vi "Periodic Tasks.vi"(8 "error in":errorcluster) -> ()   [LabVIEW 2013]
doc: "This VI runs in parallel to other tasks. It can contain as many user-defined periodic loops as you need. These can carry out PID or other sorts of timed response."
uses:
  RefnameEnum.ctl
  CatchAction.ctl
  CollectorWrapAction.ctl
  ShooterWrapperAction.ctl
  DoubleSolenoidAction.ctl
  SingleSolenoidAction.ctl
  <vilib>/Rock Robotics/SystemInterfaces/Utilities/FPGA_UtilitiesLED Source.ctl
  <vilib>/Rock Robotics/SystemInterfaces/Utilities/FPGA_UtilitiesLED State.ctl
  TankDriveAction.ctl
  SonarAction.ctl
  AutoAlignMode.ctl
  <vilib>/Rock Robotics/WPI/Compressor/WPI_CompressorGetSetRefNum.vi
  Robot Global Data.vi
panel:
  out "AutoDistanceWrapperIterations":i32=4516
  out "AutoDistanceWrapperTimer":u32=21
  in  "Slowdown":dbl=12.0 format="%#_13g"
  in  "Brake":dbl=6.0 format="%#_13g"
  in  "DesiredDistance":dbl=36.0 format="%#_13g"
  out "CatcherWrapperIterations":i32=1817
  out "CatcherWrapperTimer":u32=50
  out "CollectorWrapperTimer":u32=50
  out "CollectorWrapperIterations":i32=1817
  out "ShooterWrapperIterations":i32=1813
  out "ShooterWrapperTimer":u32=50
  out "CollectorIterations":i32=1817
  out "ClapperIterations":i32=1817
  out "RollerPneumaticIterations":i32=1817
  out "RollerMotorIterations":i32=1817
  out "FiringCylinderIterations":i32=1817
  out "KickerIterations":i32=1817
  out "SonicShifterIterations":i32=1817
  out "TankDriveIterations":i32=4509
  out "Collector Timer":u32=50
  out "Clapper Timer":u32=50
  out "Roller Pneumatic Timer":u32=50
  out "Firing Cylinder Timer":u32=50
  out "Sonic Shifter Timer":u32=50
  out "Kicker Timer":u32=50
  out "Roller Motor Timer":u32=50
  out "Tank Drive Timer":u32=21
  # "CATCH"
  # "SHOOTER WRAP"
  # "SONIC SHIFTER"
  # "TANK DRIVE"
  # "COLLECTOR WRAP"
  # "KICKER"
  # "ROLLER MOTOR"
  # "COLLECTOR ARM"
  # "FIRING CYLINDERS"
  # "AUTODISTANCE"
  # "ROLLER PNEUMATIC"
  # "CLAPPER"
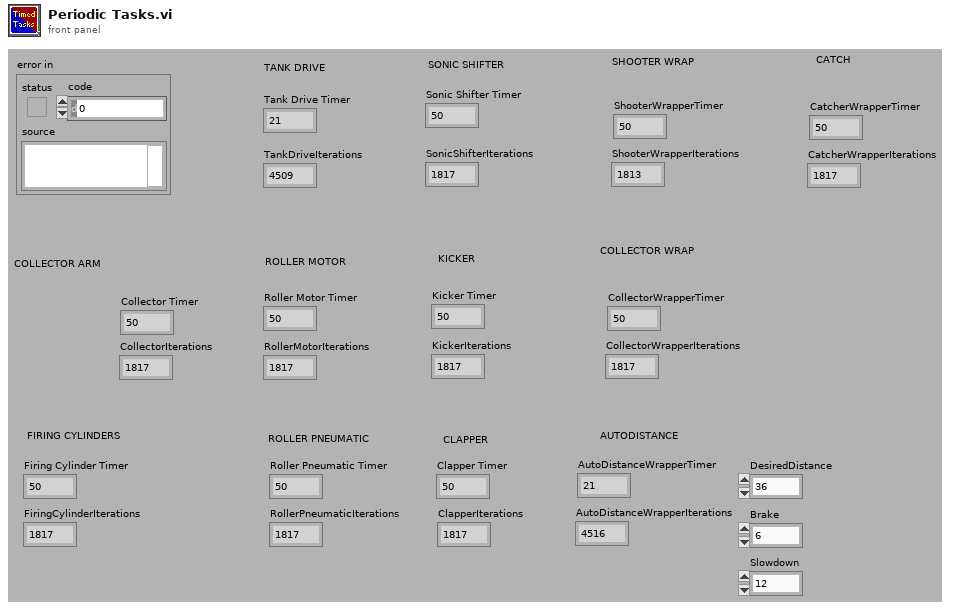
[diagram p1: front panel]
types:
  T1 = typedef "ShooterWrapperAction.ctl" = enum16{"Init", "CollectorDown", "CollectorUp"}
  T2 = typedef "CatchAction.ctl" = enum16{"PreCatch", "Catch", "Stop"}
  T3 = typedef "DoubleSolenoidAction.ctl" = enum16{"Init", "Middle", "In", "Out"}
  T4 = typedef "CollectorAction.ctl" = enum16{"Init", "Raise", "Lower", "Stop", "GetStatus"}
  T5 = typedef "CollectorWrapAction.ctl" = enum16{"PreCollect", "Collect", "Stop"}
  T6 = typedef "SingleSolenoidAction.ctl" = enum16{"Init", "SetState", "Disable"}
  T7 = typedef "TankDriveAction.ctl" = enum16{"Init", "LinearDrive", "SetValue", "Disable"}
  T8 = typedef "AutoAlignMode.ctl" = enum16{"Fullspeed", "Linear"}
  T9 = typedef "SonarAction.ctl" = enum16{"Init", "ReadValue", "Disable"}
  T10 = typedef "FPGA_UtilitiesLED State.ctl" = enum16{"Off", "On", "Toggle"}
  T11 = typedef "FPGA_UtilitiesLED Source.ctl" = enum16{"User LED", "FPGA LED"}
  T12 = typedef "RefnameEnum.ctl" = enum16{"TankDrive", "Controller1", "Controller2", "SonicShifter", "Compressor"}
  T13 = typedef "WPI_CompressorDevRef.ctl" = cluster{"DevStatus":errorcluster, "DigitalInputDevRef":T14, "RelayDevRef":T17}
  T14 = typedef "WPI_DigitalInputDevRef.ctl" = cluster{"DevStatus":errorcluster, "DIO Channel":T15, "Digital Module":T16}
  T15 = typedef "FPGA_DIOChannel.ctl" = enum8{"DIO 1", "DIO 2", "DIO 3", "DIO 4", "DIO 5", "DIO 6", "DIO 7", "DIO 8", "DIO 9", "DIO 10", "DIO 11", "DIO 12", "DIO 13", "DIO 14", "Invalid"}
  T16 = typedef "FPGA_TypedefDigitalModule.ctl" = enum16{"Digital Module 1", "Digital Module 2"}
  T17 = typedef "WPI_RelayDevRef.ctl" = cluster{"DevStatus":errorcluster, "Relay Channel":T18, "Digital Module":T16, "Relay Direction":T19}
  T18 = typedef "FPGA_DIORelayChannel.ctl" = enum8{"Relay 1", "Relay 2", "Relay 3", "Relay 4", "Relay 5", "Relay 6", "Relay 7", "Relay 8", "Invalid"}
  T19 = typedef "WPI_RelayDirection.ctl" = enum16{"Both directions", "Forward only", "Reverse only"}
  T20 = typedef "RollerAction.ctl" = enum16{"Init", "Off", "Forward", "Reverse"}
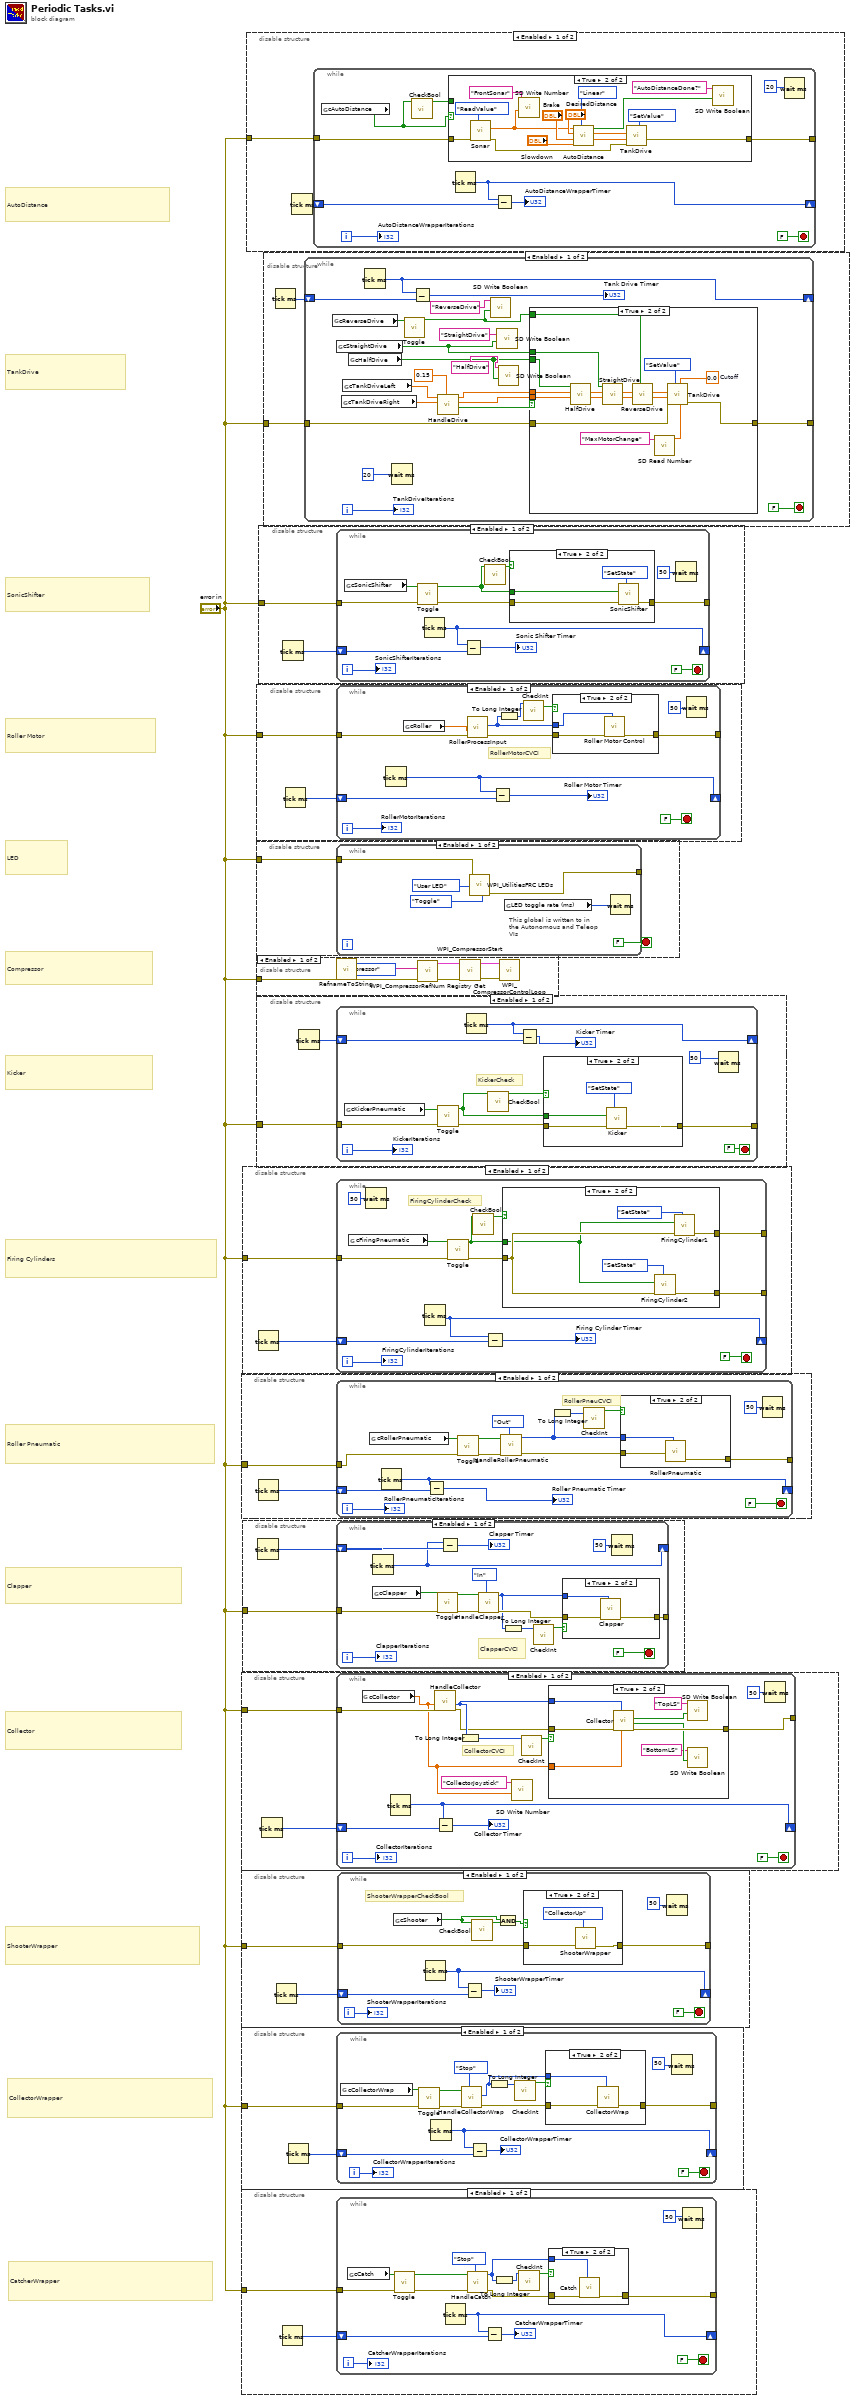
[diagram p0: block diagram]
diagram:
  # "AutoDistance"
  # "CatcherWrapper"
  # "CollectorWrapper"
  # "ShooterWrapper"
  # "Collector"
  # "Clapper"
  # "Roller Pneumatic"
  # "Firing Cylinders"
  # "Kicker"
  # "Compressor"
  # "Roller Motor"
  # "SonicShifter"
  # "LED"
  # "TankDrive"
  n1 = disable-structure shown="Enabled" {
    disable-tunnel: "error in" -> [w3 _]
    frame Enabled {
      n2 = Tick Count (ms)() -> (millisecond timer value=w2:u32)
      n3 = while {
        tunnel: w3 -> [w10]
        shift-right: [w11] -> _
        shift-left: w2 -> [w12]
        tunnel: [w9] -> _
        i -> [w7]
        stop <- FALSE stop-if-true
        # "ShooterWrapperCheckBool"
        n4 = global read "Robot Global Data.vi" "cShooter"() -> (w4:bool)
        n5 = Tick Count (ms)() -> (millisecond timer value=w11:u32)
        n6 = Subtract(x=w11, y=w12) -> (x-y=→"ShooterWrapperTimer":u32)
        n7 = call "CheckBool.vi"("Input Boolean"=w4) -> ("Boolean Changed?"=w6:bool)  [unwired: 10 in]
        n8 = And(x=w4, y=w6) -> (x .and. y?=w5:bool)
        n9 = case shown="True" w5 {
          tunnel: w10 -> [w15 w18]
          tunnel: [w15 w17] -> w9
          frame False {
          }
          frame True {
            n10 = call "ShooterWrapper.vi"("Action"=ShooterWrapperAction."CollectorUp", "error in"=w18) -> ("error out"=w17:errorcluster)  [unwired: 8 in]
          }
        }
        n11 = Wait (ms)(milliseconds to wait=u32 50) -> ()  [unwired: 1 out]
        "ShooterWrapperIterations" <- w7
      }
    }
    frame Disabled {
    }
  }
  n12 = disable-structure shown="Enabled" {
    disable-tunnel: "error in" -> [w20 _]
    frame Enabled {
      n13 = Tick Count (ms)() -> (millisecond timer value=w19:u32)
      n14 = while {
        tunnel: w20 -> [w36]
        tunnel: [w33] -> _
        shift-right: [w28] -> _
        shift-left: w19 -> [w29]
        i -> [w30]
        stop <- FALSE stop-if-true
        n15 = global read "Robot Global Data.vi" "cCatch"() -> (w35:bool)
        n16 = call "Toggle.vi"("error in"=w36, "RawInput"=w35) -> ("error out"=w26:errorcluster, "ToggleState"=w22:bool)  [unwired: 8 in]
        n17 = Tick Count (ms)() -> (millisecond timer value=w28:u32)
        n18 = call "HandleCatch.vi"("InitState"=CatchAction."Stop", "error in (no error)"=w26, "Toggle?"=w22) -> ("error out"=w25:errorcluster, "State"=w23:T2)  [unwired: 7 in]
        n19 = Subtract(x=w28, y=w29) -> (x-y=→"CatcherWrapperTimer":u32)
        n20 = To Long Integer(number=w23) -> (32bit integer=w24:i32)
        n21 = call "CheckInt.vi"("Integer"=w24) -> ("Changed?"=w34:bool)  [unwired: 10 in]
        n22 = case shown="True" w34 {
          tunnel: w25 -> [w37 w40]
          tunnel: [w37 w39] -> w33
          tunnel: w23 -> [_ w38]
          frame False {
          }
          frame True {
            n23 = call "Catch.vi"("Action"=w38, "error in (no error)"=w40) -> ("error out"=w39:errorcluster)  [unwired: 9 in]
          }
        }
        n24 = Wait (ms)(milliseconds to wait=u32 50) -> ()  [unwired: 1 out]
        "CatcherWrapperIterations" <- w30
      }
    }
    frame Disabled {
    }
  }
  n25 = disable-structure shown="Enabled" {
    disable-tunnel: "error in" -> [w42 _]
    frame Enabled {
      n26 = Tick Count (ms)() -> (millisecond timer value=w41:u32)
      n27 = while {
        tunnel: w42 -> [w46]
        shift-right: [w55] -> _
        shift-left: w41 -> [w54]
        tunnel: [w48] -> _
        i -> [w47]
        stop <- FALSE stop-if-true
        # "RollerPneuCVCI"
        n28 = global read "Robot Global Data.vi" "cRollerPneumatic"() -> (w44:bool)
        n29 = Tick Count (ms)() -> (millisecond timer value=w55:u32)
        n30 = Subtract(x=w55, y=w54) -> (x-y=→"Roller Pneumatic Timer":u32)
        n31 = call "Toggle.vi"("error in"=w46, "RawInput"=w44) -> ("error out"=w45:errorcluster, "ToggleState"=w43:bool)  [unwired: 8 in]
        n32 = call "HandleRollerPneumatic.vi"("InitState"=DoubleSolenoidAction."Out", "error in (no error)"=w45, "Toggle?"=w43) -> ("error out"=w49:errorcluster, "State"=w50:T3)  [unwired: 7 in]
        n33 = To Long Integer(number=w50) -> (32bit integer=w52:i32)
        n34 = call "CheckInt.vi"("Integer"=w52) -> ("Changed?"=w51:bool)  [unwired: 10 in]
        n35 = case shown="True" w51 {
          tunnel: w50 -> [_ w62]
          tunnel: w49 -> [w59 w61]
          tunnel: [w59 w60] -> w48
          frame False {
          }
          frame True {
            n36 = call "RollerPneumatic.vi"("State"=w62, "Error in"=w61) -> ("Error out"=w60:errorcluster)  [unwired: 9 in]
          }
        }
        n37 = Wait (ms)(milliseconds to wait=u32 50) -> ()  [unwired: 1 out]
        "RollerPneumaticIterations" <- w47
      }
    }
    frame Disabled {
    }
  }
  n38 = disable-structure shown="Enabled" {
    disable-tunnel: "error in" -> [w64 _]
    frame Enabled {
      n39 = Tick Count (ms)() -> (millisecond timer value=w63:u32)
      n40 = while {
        tunnel: w64 -> [w77]
        shift-right: [w74] -> _
        shift-left: w63 -> [w75]
        tunnel: [w68] -> _
        i -> [w67]
        stop <- FALSE stop-if-true
        # "CollectorCVCI"
        n41 = global read "Robot Global Data.vi" "cCollector"() -> (w65:dbl)
        n42 = Tick Count (ms)() -> (millisecond timer value=w74:u32)
        n43 = call "HandleCollector.vi"("error in"=w77, "JoystickValue"=w65) -> ("error out"=w69:errorcluster, "CollectorEnum Input"=w70:T4)  [unwired: 8 in]
        n44 = Subtract(x=w74, y=w75) -> (x-y=→"Collector Timer":u32)
        n45 = To Long Integer(number=w70) -> (32bit integer=w72:i32)
        n46 = call <vilib>:"SD Write Number.vi"("Numeric"=w65, "Name"="CollectorJoystick") -> ()  [unwired: 8 in, 2 out]
        n47 = call "CheckInt.vi"("Integer"=w72) -> ("Changed?"=w71:bool)  [unwired: 10 in]
        n48 = case shown="True" w71 {
          tunnel: w70 -> [_ w87]
          tunnel: w69 -> [w79 w86]
          tunnel: [w79 w85] -> w68
          tunnel: w65 -> [_ w80]
          frame False {
          }
          frame True {
            n49 = call "Collector.vi"("MotorSpeed"=w80, "Action"=w87, "Error in"=w86) -> ("Error out"=w85:errorcluster, "Lower Triggered?"=w83:bool, "Upper Triggered?"=w84:bool)  [unwired: 6 in]
            n50 = call <vilib>:"SD Write Boolean.vi"("Boolean"=w84, "Name"="TopLS") -> ()  [unwired: 8 in, 2 out]
            n51 = call <vilib>:"SD Write Boolean.vi"("Boolean"=w83, "Name"="BottomLS") -> ()  [unwired: 8 in, 2 out]
          }
        }
        n52 = Wait (ms)(milliseconds to wait=u32 50) -> ()  [unwired: 1 out]
        "CollectorIterations" <- w67
      }
    }
    frame Disabled {
    }
  }
  n53 = disable-structure shown="Enabled" {
    disable-tunnel: "error in" -> [w89 _]
    frame Enabled {
      n54 = Tick Count (ms)() -> (millisecond timer value=w88:u32)
      n55 = while {
        tunnel: w89 -> [w98]
        shift-right: [w102] -> _
        shift-left: w88 -> [w103]
        tunnel: [w101] -> _
        i -> [w99]
        stop <- FALSE stop-if-true
        n56 = global read "Robot Global Data.vi" "cCollectorWrap"() -> (w97:bool)
        n57 = call "Toggle.vi"("error in"=w98, "RawInput"=w97) -> ("error out"=w96:errorcluster, "ToggleState"=w94:bool)  [unwired: 8 in]
        n58 = Tick Count (ms)() -> (millisecond timer value=w102:u32)
        n59 = call "HandleCollectorWrap.vi"("InitState"=CollectorWrapAction."Stop", "error in (no error)"=w96, "Toggle?"=w94) -> ("error out"=w93:errorcluster, "State"=w90:T5)  [unwired: 7 in]
        n60 = Subtract(x=w102, y=w103) -> (x-y=→"CollectorWrapperTimer":u32)
        n61 = To Long Integer(number=w90) -> (32bit integer=w91:i32)
        n62 = call "CheckInt.vi"("Integer"=w91) -> ("Changed?"=w92:bool)  [unwired: 10 in]
        n63 = case shown="True" w92 {
          tunnel: [w106 w109] -> w101
          tunnel: w93 -> [w106 w108]
          tunnel: w90 -> [_ w107]
          frame False {
          }
          frame True {
            n64 = call "CollectorWrap.vi"("Action"=w107, "error in"=w108) -> ("error out"=w109:errorcluster)  [unwired: 9 in]
          }
        }
        n65 = Wait (ms)(milliseconds to wait=u32 50) -> ()  [unwired: 1 out]
        "CollectorWrapperIterations" <- w99
      }
    }
    frame Disabled {
    }
  }
  n66 = disable-structure shown="Enabled" {
    disable-tunnel: "error in" -> [w111 _]
    frame Enabled {
      n67 = Tick Count (ms)() -> (millisecond timer value=w110:u32)
      n68 = while {
        tunnel: w111 -> [w116]
        shift-right: [w122] -> _
        shift-left: w110 -> [w121]
        tunnel: [w119] -> _
        tunnel: [w118] -> _
        i -> [w112]
        stop <- FALSE stop-if-true
        # "FiringCylinderCheck"
        n69 = global read "Robot Global Data.vi" "cFiringPneumatic"() -> (w117:bool)
        n70 = Wait (ms)(milliseconds to wait=u32 50) -> ()  [unwired: 1 out]
        n71 = Tick Count (ms)() -> (millisecond timer value=w122:u32)
        n72 = call "Toggle.vi"("error in"=w116, "RawInput"=w117) -> ("error out"=w115:errorcluster, "ToggleState"=w113:bool)  [unwired: 8 in]
        n73 = call "CheckBool.vi"("Input Boolean"=w113) -> ("Boolean Changed?"=w114:bool)  [unwired: 10 in]
        n74 = Subtract(x=w122, y=w121) -> (x-y=→"Firing Cylinder Timer":u32)
        n75 = case shown="True" w114 {
          tunnel: w115 -> [w125 w127]
          tunnel: [w125 w129] -> w119
          tunnel: [w125 w128] -> w118
          tunnel: w113 -> [_ w126]
          frame False {
          }
          frame True {
            n76 = call "FiringCylinder2.vi"("Action"=SingleSolenoidAction."SetState", "error in (no error)"=w127, "Actuate?"=w126) -> ("error out"=w128:errorcluster)  [unwired: 8 in]
            n77 = call "FiringCylinder1.vi"("Action"=SingleSolenoidAction."SetState", "error in (no error)"=w127, "Actuate?"=w126) -> ("error out"=w129:errorcluster)  [unwired: 8 in]
          }
        }
        "FiringCylinderIterations" <- w112
      }
    }
    frame Disabled {
    }
  }
  n78 = disable-structure shown="Enabled" {
    disable-tunnel: "error in" -> [w133 _]
    frame Enabled {
      n79 = Tick Count (ms)() -> (millisecond timer value=w132:u32)
      n80 = while {
        tunnel: w133 -> [w138]
        shift-right: [w134] -> _
        shift-left: w132 -> [w135]
        tunnel: [w144] -> _
        i -> [w140]
        stop <- FALSE stop-if-true
        # "ClapperCVCI"
        n81 = Tick Count (ms)() -> (millisecond timer value=w134:u32)
        n82 = global read "Robot Global Data.vi" "cClapper"() -> (w139:bool)
        n83 = call "Toggle.vi"("error in"=w138, "RawInput"=w139) -> ("error out"=w137:errorcluster, "ToggleState"=w136:bool)  [unwired: 8 in]
        n84 = Subtract(x=w134, y=w135) -> (x-y=→"Clapper Timer":u32)
        n85 = call "HandleClapper.vi"("InitState"=DoubleSolenoidAction."In", "error in (no error)"=w137, "Toggle?"=w136) -> ("error out"=w145:errorcluster, "State"=w142:T3)  [unwired: 7 in]
        n86 = To Long Integer(number=w142) -> (32bit integer=w143:i32)
        n87 = call "CheckInt.vi"("Integer"=w143) -> ("Changed?"=w141:bool)  [unwired: 10 in]
        n88 = case shown="True" w141 {
          tunnel: w142 -> [_ w153]
          tunnel: w145 -> [w150 w152]
          tunnel: [w150 w151] -> w144
          frame False {
          }
          frame True {
            n89 = call "Clapper.vi"("State"=w153, "Error in"=w152) -> ("Error out"=w151:errorcluster)  [unwired: 9 in]
          }
        }
        n90 = Wait (ms)(milliseconds to wait=u32 50) -> ()  [unwired: 1 out]
        "ClapperIterations" <- w140
      }
    }
    frame Disabled {
    }
  }
  n91 = disable-structure shown="Enabled" {
    disable-tunnel: "error in" -> [w155 _]
    frame Enabled {
      n92 = Tick Count (ms)() -> (millisecond timer value=w154:u32)
      n93 = while {
        tunnel: w155 -> [w165]
        tunnel: [w164] -> _
        shift-right: [w159] -> _
        shift-left: w154 -> [w160]
        i -> [w161]
        stop <- FALSE stop-if-true
        n94 = global read "Robot Global Data.vi" "cAutoDistance"() -> (w157:bool)
        n95 = call "CheckBool.vi"("Input Boolean"=w157) -> ("Boolean Changed?"=w156:bool)  [unwired: 10 in]
        n96 = case shown="True" w157 {
          tunnel: w165 -> [w168 w184]
          tunnel: [w167 w181] -> w164
          tunnel: w156 -> [w166 _]
          frame False {
            n97 = case shown="True" w166 {
              tunnel: w168 -> [w169 w173]
              tunnel: [w169 w172] -> w167
              frame False {
              }
              frame True {
                w171 = 0.0 ("LeftDesired")
                n98 = call "TankDrive.vi"("DriveAction"=TankDriveAction."SetValue", "error in (no error)"=w173, "RightDesired"=w171, "LeftDesired"=w171) -> ("error out"=w172:errorcluster)  [unwired: 6 in, 1 out]
              }
            }
          }
          frame True {
            n99 = call "Sonar.vi"("Action"=SonarAction."ReadValue", "error in (no error)"=w184) -> ("error out"=w178:errorcluster, "distance"=w180:dbl)  [unwired: 8 in]
            n100 = call <vilib>:"SD Write Number.vi"("Numeric"=w180, "Name"="FrontSonar") -> ()  [unwired: 8 in, 2 out]
            n101 = call "AutoDistance.vi"("Mode"=AutoAlignMode."Linear", "Slowdown"="Slowdown", "Brake"="Brake", "DesiredDistance"="DesiredDistance", "CurrentDistance"=w180) -> ("TankDriveRight"=w174:dbl, "TankDriveLeft"=w175:dbl, "Finished"=w177:bool)  [unwired: 4 in]
            n102 = call "TankDrive.vi"("DriveAction"=TankDriveAction."SetValue", "error in (no error)"=w178, "RightDesired"=w174, "LeftDesired"=w175) -> ("error out"=w181:errorcluster)  [unwired: 6 in, 1 out]
            n103 = call <vilib>:"SD Write Boolean.vi"("Boolean"=w177, "Name"="AutoDistanceDone?") -> ()  [unwired: 8 in, 2 out]
          }
        }
        n104 = Tick Count (ms)() -> (millisecond timer value=w159:u32)
        n105 = Subtract(x=w159, y=w160) -> (x-y=→"AutoDistanceWrapperTimer":u32)
        n106 = Wait (ms)(milliseconds to wait=u32 20) -> ()  [unwired: 1 out]
        "AutoDistanceWrapperIterations" <- w161
      }
    }
    frame Disabled {
    }
  }
  n107 = disable-structure shown="Enabled" {
    disable-tunnel: "error in" -> [w189 _]
    frame Enabled {
      n108 = while {
        tunnel: w189 -> [w191]
        tunnel: [w190] -> _
        stop <- FALSE stop-if-true
        # "This global is written to in the Autonomous and Teleop VIs"
        n109 = call <vilib>:"WPI_UtilitiesFRC LEDs.vi"("error in (no error)"=w191, "State"=FPGA_UtilitiesLED_State."Toggle", "LED Type"=FPGA_UtilitiesLED_Source."User LED") -> ("error out"=w190:errorcluster)  [unwired: 8 out]
        n110 = global read "Robot Global Data.vi" "LED toggle rate (ms)"() -> (w192:u32)
        n111 = Wait (ms)(milliseconds to wait=w192) -> ()  [unwired: 1 out]
      }
    }
    frame Disabled {
    }
  }
  n112 = disable-structure shown="Enabled" {
    disable-tunnel: "error in" -> [w202 _]
    frame Enabled {
      n113 = call "RefnameToString.vi"("Enum"=RefnameEnum."Compressor") -> ("Refname"=w199:string)
      n114 = call <vilib>:"WPI_CompressorRefNum Registry Get.vi"("error in (no error)"=w202, "refnum name"=w199) -> ("error out"=w201:errorcluster, "CompressorDevRef"=w197:T13)  [unwired: 8 in]
      n115 = call <vilib>:"WPI_CompressorStart.vi"("error in (no error)"=w201, "CompressorDevRef"=w197) -> ("error out"=w200:errorcluster, "CompressorDevRef"=w196:T13)  [unwired: 8 in]
      n116 = call <vilib>:"WPI_CompressorControlLoop.vi"("error in (no error)"=w200, "CompressorDevRef"=w196) -> ()  [unwired: 10 in]
    }
    frame Disabled {
    }
  }
  n117 = disable-structure shown="Enabled" {
    disable-tunnel: "error in" -> [w204 _]
    frame Enabled {
      n118 = Tick Count (ms)() -> (millisecond timer value=w203:u32)
      n119 = while {
        tunnel: w204 -> [w215]
        shift-right: [w213] -> _
        shift-left: w203 -> [w211]
        tunnel: [w207] -> _
        i -> [w205]
        stop <- FALSE stop-if-true
        # "RollerMotorCVCI"
        n120 = Tick Count (ms)() -> (millisecond timer value=w213:u32)
        n121 = global read "Robot Global Data.vi" "cRoller"() -> (w214:dbl)
        n122 = call "RollerProcessInput.vi"("error in"=w215, "JoystickValue"=w214) -> ("error out"=w208:errorcluster, "StateOut"=w206:T20)  [unwired: 8 in]
        n123 = Subtract(x=w213, y=w211) -> (x-y=→"Roller Motor Timer":u32)
        n124 = To Long Integer(number=w206) -> (32bit integer=w210:i32)
        n125 = call "CheckInt.vi"("Integer"=w210) -> ("Changed?"=w209:bool)  [unwired: 10 in]
        n126 = case shown="True" w209 {
          tunnel: w206 -> [_ w221]
          tunnel: w208 -> [w218 w220]
          tunnel: [w218 w219] -> w207
          frame False {
          }
          frame True {
            n127 = call "Roller Motor Control.vi"("Action"=w221, "Error in"=w220) -> ("Error out"=w219:errorcluster)  [unwired: 9 in]
          }
        }
        n128 = Wait (ms)(milliseconds to wait=u32 50) -> ()  [unwired: 1 out]
        "RollerMotorIterations" <- w205
      }
    }
    frame Disabled {
    }
  }
  n129 = disable-structure shown="Enabled" {
    disable-tunnel: "error in" -> [w223 _]
    frame Enabled {
      n130 = Tick Count (ms)() -> (millisecond timer value=w222:u32)
      n131 = while {
        tunnel: w223 -> [w229]
        shift-right: [w231] -> _
        shift-left: w222 -> [w233]
        tunnel: [w230] -> _
        i -> [w224]
        stop <- FALSE stop-if-true
        # "KickerCheck"
        n132 = global read "Robot Global Data.vi" "cKickerPneumatic"() -> (w227:bool)
        n133 = call "Toggle.vi"("error in"=w229, "RawInput"=w227) -> ("error out"=w228:errorcluster, "ToggleState"=w225:bool)  [unwired: 8 in]
        n134 = Tick Count (ms)() -> (millisecond timer value=w231:u32)
        n135 = call "CheckBool.vi"("Input Boolean"=w225) -> ("Boolean Changed?"=w226:bool)  [unwired: 10 in]
        n136 = Subtract(x=w231, y=w233) -> (x-y=→"Kicker Timer":u32)
        n137 = case shown="True" w226 {
          tunnel: w228 -> [w236 w238]
          tunnel: [w236 w239] -> w230
          tunnel: w225 -> [_ w237]
          frame False {
          }
          frame True {
            n138 = call "Kicker.vi"("Action"=SingleSolenoidAction."SetState", "error in (no error)"=w238, "Actuate?"=w237) -> ("error out"=w239:errorcluster)  [unwired: 8 in]
          }
        }
        n139 = Wait (ms)(milliseconds to wait=u32 50) -> ()  [unwired: 1 out]
        "KickerIterations" <- w224
      }
    }
    frame Disabled {
    }
  }
  n140 = disable-structure shown="Enabled" {
    disable-tunnel: "error in" -> [w242 _]
    frame Enabled {
      n141 = Tick Count (ms)() -> (millisecond timer value=w241:u32)
      n142 = while {
        tunnel: w242 -> [w247]
        shift-right: [w251] -> _
        shift-left: w241 -> [w252]
        tunnel: [w249] -> _
        i -> [w244]
        stop <- FALSE stop-if-true
        n143 = global read "Robot Global Data.vi" "cSonicShifter"() -> (w248:bool)
        n144 = call "Toggle.vi"("error in"=w247, "RawInput"=w248) -> ("error out"=w246:errorcluster, "ToggleState"=w243:bool)  [unwired: 8 in]
        n145 = Tick Count (ms)() -> (millisecond timer value=w251:u32)
        n146 = Subtract(x=w251, y=w252) -> (x-y=→"Sonic Shifter Timer":u32)
        n147 = call "CheckBool.vi"("Input Boolean"=w243) -> ("Boolean Changed?"=w245:bool)  [unwired: 10 in]
        n148 = case shown="True" w245 {
          tunnel: [w255 w258] -> w249
          tunnel: w246 -> [w255 w257]
          tunnel: w243 -> [_ w256]
          frame False {
          }
          frame True {
            n149 = call "SonicShifter.vi"("Action"=SingleSolenoidAction."SetState" ("Mode"), "error in (no error)"=w257, "Actuate?"=w256) -> ("error out"=w258:errorcluster)  [unwired: 8 in]
          }
        }
        n150 = Wait (ms)(milliseconds to wait=u32 50) -> ()  [unwired: 1 out]
        "SonicShifterIterations" <- w244
      }
    }
    frame Disabled {
    }
  }
  n151 = disable-structure shown="Enabled" {
    disable-tunnel: "error in" -> [w261 _]
    frame Enabled {
      n152 = Tick Count (ms)() -> (millisecond timer value=w260:u32)
      n153 = while {
        tunnel: w261 -> [w272]
        shift-right: [w281] -> _
        shift-left: w260 -> [w280]
        tunnel: [w273] -> _
        i -> [w269]
        stop <- FALSE stop-if-true
        n154 = global read "Robot Global Data.vi" "cReverseDrive"() -> (w268:bool)
        n155 = global read "Robot Global Data.vi" "cStraightDrive"() -> (w265:bool)
        n156 = global read "Robot Global Data.vi" "cTankDriveRight"() -> (w278:dbl)
        n157 = global read "Robot Global Data.vi" "cTankDriveLeft"() -> (w277:dbl)
        n158 = global read "Robot Global Data.vi" "cHalfDrive"() -> (w264:bool)
        n159 = Tick Count (ms)() -> (millisecond timer value=w281:u32)
        n160 = Wait (ms)(milliseconds to wait=u32 20) -> ()  [unwired: 1 out]
        n161 = call "Toggle.vi"("RawInput"=w268) -> ("ToggleState"=w262:bool)  [unwired: 9 in, 1 out]
        n162 = Subtract(x=w281, y=w280) -> (x-y=→"Tank Drive Timer":u32)
        n163 = call "HandleDrive.vi"("Deadzone"=0.15, "RightMotor"=w278, "LeftMotor"=w277) -> ("Enqueue?"=w276:bool, "RightMotor"=w274:dbl, "LeftMotor"=w275:dbl)  [unwired: 6 in]
        n164 = call <vilib>:"SD Write Boolean.vi"("Boolean"=w262, "Name"="ReverseDrive") -> ()  [unwired: 8 in, 2 out]
        n165 = call <vilib>:"SD Write Boolean.vi"("Boolean"=w265, "Name"="StraightDrive") -> ()  [unwired: 8 in, 2 out]
        n166 = call <vilib>:"SD Write Boolean.vi"("Boolean"=w264, "Name"="HalfDrive") -> ()  [unwired: 8 in, 2 out]
        n167 = case shown="True" w276 {
          tunnel: w275 -> [_ w292]
          tunnel: w274 -> [_ w291]
          tunnel: [w283 w290] -> w273
          tunnel: w272 -> [w283 w289]
          tunnel: w262 -> [_ w286]
          tunnel: w264 -> [_ w285]
          tunnel: w265 -> [_ w284]
          frame False {
          }
          frame True {
            w299 = 0.0  # Cutoff
            n168 = call "HalfDrive.vi"("RightDrive in"=w291, "LeftDrive in"=w292, "HalfDrive"=w285) -> ("RightDrive out"=w298:dbl, "LeftDrive out"=w297:dbl)  [unwired: 7 in]
            n169 = call "StraightDrive.vi"("RightDrive in"=w298, "LeftDrive in"=w297, "StraightDrive"=w284) -> ("RightDrive out"=w295:dbl, "LeftDrive out"=w296:dbl)  [unwired: 7 in]
            n170 = call "ReverseDrive.vi"("cReverseDrive"=w286, "Right"=w295, "Left"=w296) -> ("Right"=w293:dbl, "Left"=w294:dbl)  [unwired: 7 in]
            n171 = call <vilib>:"SD Read Number.vi"("Name"="MaxMotorChange") -> ("Numeric"=w287:dbl)  [unwired: 8 in, 2 out]
            n172 = call "TankDrive.vi"("MaxMotorChangeForward"=w287, "Cutoff"=w299, "DriveAction"=TankDriveAction."SetValue", "error in (no error)"=w289, "RightDesired"=w293, "LeftDesired"=w294) -> ("error out"=w290:errorcluster)  [unwired: 4 in, 1 out]
          }
        }
        "TankDriveIterations" <- w269
      }
    }
    frame Disabled {
    }
  }
